vi "Scheduler.vi"(1 "RampRates":T1(array[cluster]), 3 "Room Temperature":dbl, 4 "CentigradeToFahrenheit":bool, 5 "error in (no error)":errorcluster, 6 "Action":dbl, 7 "Process_REF":string, 8 "State":dbl, 9 "Machine Settings":T2, 11 "Read File":string) -> (10 "Initialized":bool, 12 "Is Valid Schedule":bool, 13 "Waveform":waveform(dbl), 14 "Path Out":path, 15 "Setpoint Profile":cluster{"Time (s)":dbl, "setpoint (C)":dbl}[](array[cluster]), 17 "Sampling Rates":dbl[](array[numeric]), 18 "New RampRates":T1(array[cluster]), 19 "error out":errorcluster)   [LabVIEW 2018]
panel:
  out "Waveform Graph":waveform(dbl)(graph)
  in  "stop":bool
  in  "Path In":path
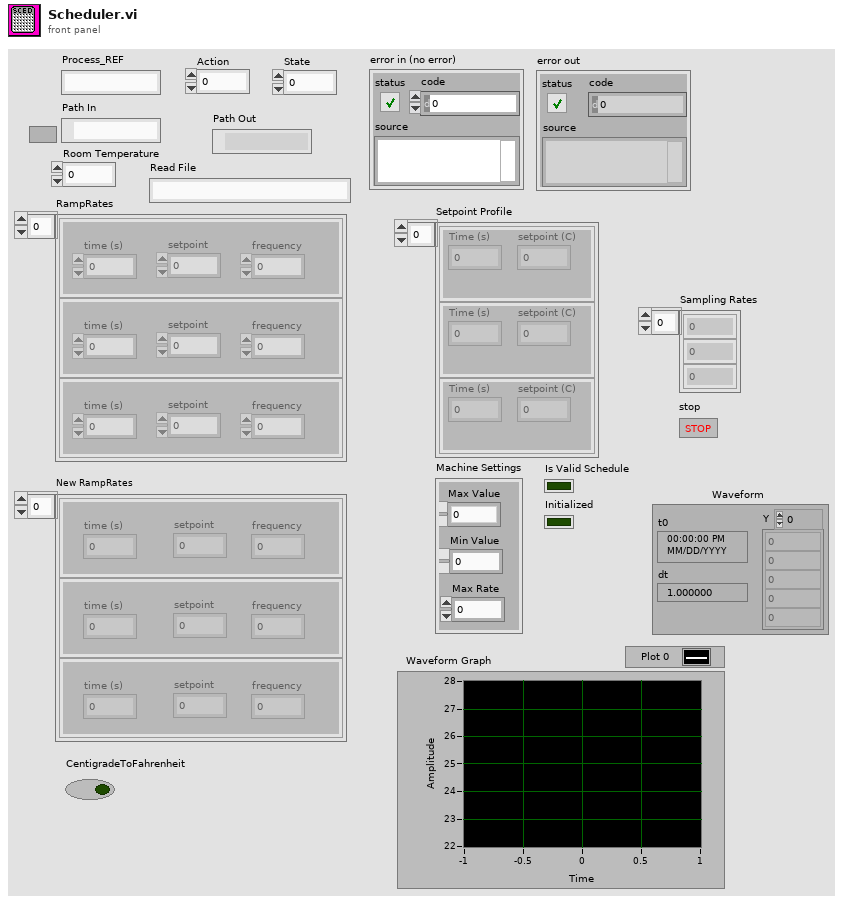
[diagram p1: front panel]
types:
  T1 = cluster{"time (s)":dbl, "setpoint ":dbl, "frequency":dbl}[]
  T2 = cluster{"Max Value":dbl, "Min Value":dbl, "Max Rate":dbl}
  T3 = cluster{"Duration (min)":dbl, "Rate (C/min) ":dbl, "Frequency (1/min)":dbl}[]
  T4 = cluster{"Duration (m)":dbl, "Rate (C/min)":dbl}[]
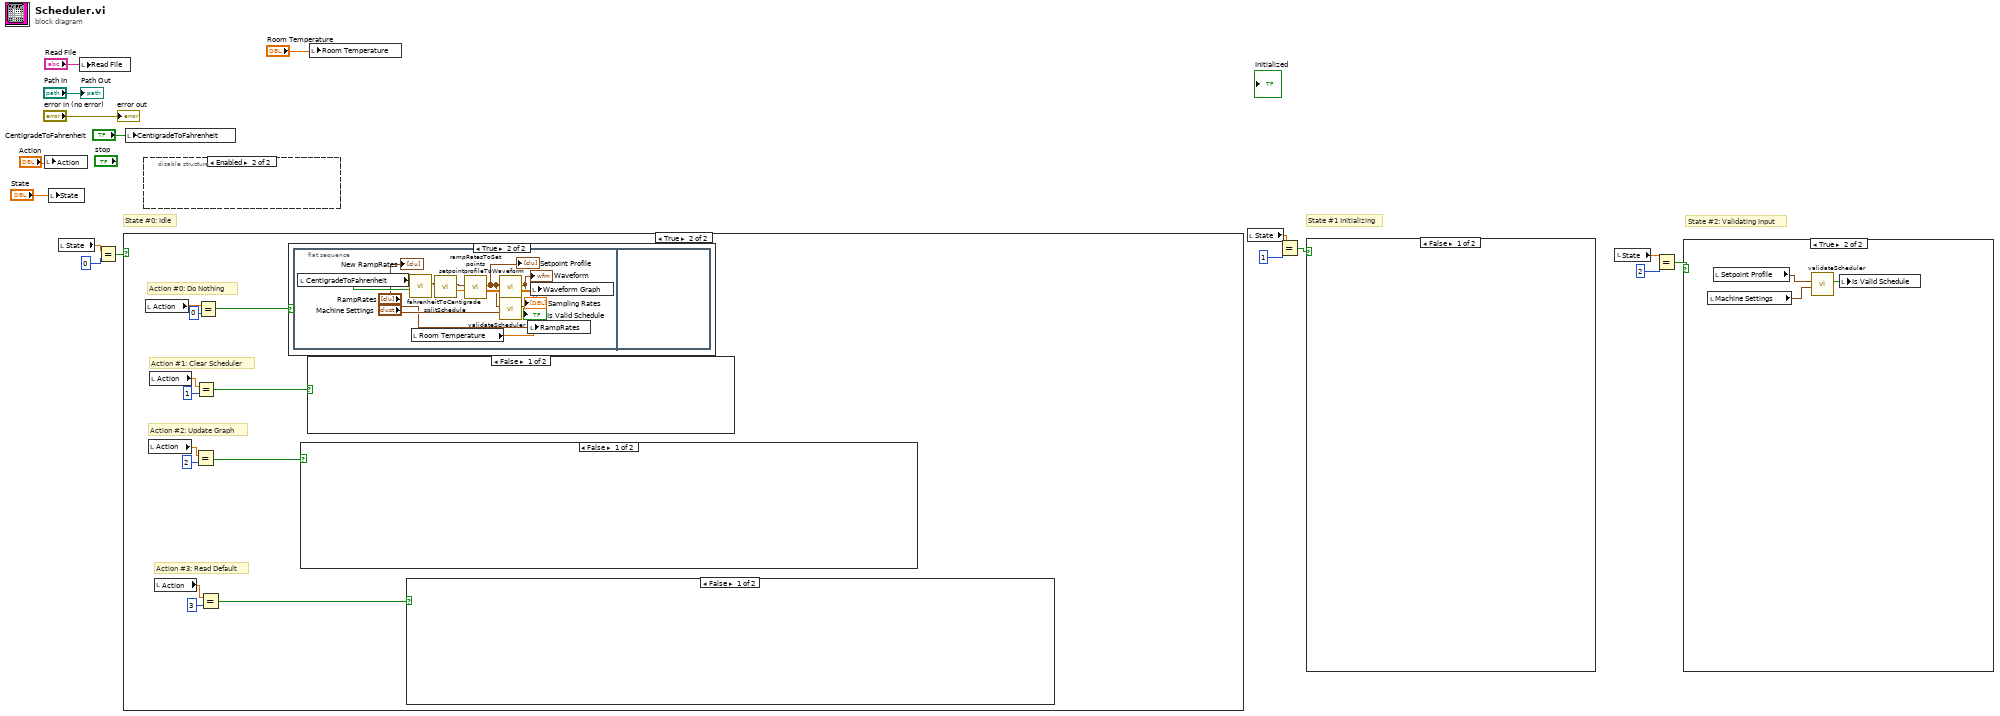
[diagram p0: block diagram]
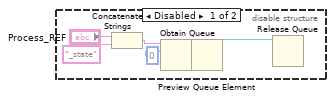
[diagram p2: hidden frame]
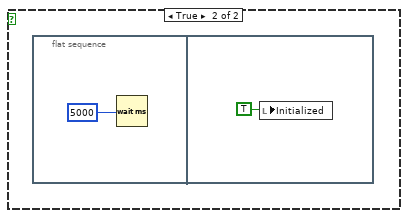
[diagram p4: hidden frame]
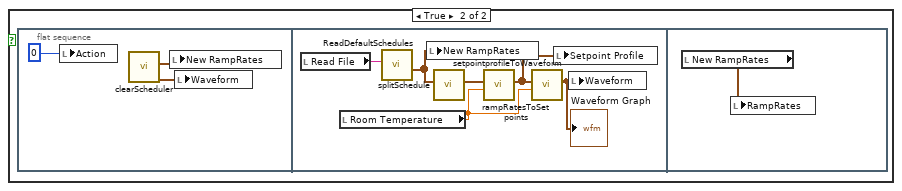
[diagram p7: hidden frame]
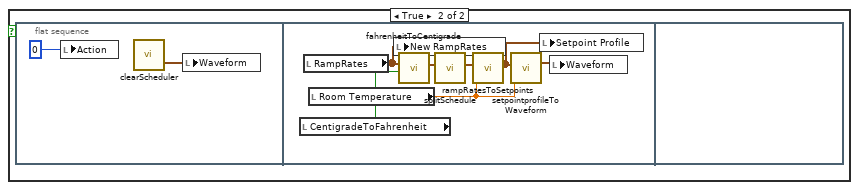
[diagram p8: hidden frame]
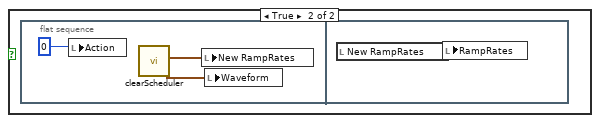
[diagram p9: hidden frame]
diagram:
  # "State #2: Validating Input"
  # "State #1 Initializing"
  # "State #0: Idle"
  n1 = local write "Action"("Action") -> ()
  n2 = local write "State"("State") -> ()
  n3 = local read "State"() -> (w11:dbl)
  n4 = local write "Read File"("Read File") -> ()
  n5 = Equal?(x=w11, y=0) -> (x = y?=w9:bool)
  n6 = case shown="True" w9 {
    frame False {
    }
    frame True {
      # "Action #0: Do Nothing"
      # "Action #3: Read Default"
      # "Action #2: Update Graph"
      # "Action #1: Clear Scheduler"
      n7 = local read "Action"() -> (w18:dbl)
      n8 = local read "Action"() -> (w24:dbl)
      n9 = local read "Action"() -> (w27:dbl)
      n10 = local read "Action"() -> (w21:dbl)
      n11 = Equal?(x=w24, y=2) -> (x = y?=w23:bool)
      n12 = Equal?(x=w27, y=1) -> (x = y?=w26:bool)
      n13 = Equal?(x=w18, y=0) -> (x = y?=w17:bool)
      n14 = Equal?(x=w21, y=3) -> (x = y?=w20:bool)
      n15 = case shown="True" w17 {
        frame False {
        }
        frame True {
          n16 = flat-sequence {
            frame #0 {
              n17 = local read "CentigradeToFahrenheit"() -> (w32:bool)
              n18 = call "fahrenheitToCentigrade.vi"("Convert?"=w32, "Schedule Before"="RampRates") -> ("Schedule After"=w33:T3)  [unwired: 9 in]
              n19 = local read "Room Temperature"() -> (w38:dbl)
              n20 = call "splitSchedule.vi"("Schedule"=w33) -> ("Sampling Rates"=→"Sampling Rates":dbl[], "Ramp Rates"=w36:T4)  [unwired: 9 in]
              n21 = call "rampRatesToSetpoints.vi"("Room Temperature"=w38, "Ramp Rates"=w36) -> ("Setpoint Profile"=w29:cluster{"Time (s)":dbl, "Setpoint (C)":dbl}[])  [unwired: 9 in]
              "Setpoint Profile" <- w29
              n22 = call "setpointprofileToWaveform.vi"("Room Temp Offset"=w38, "setpoint profile"=w29) -> ("Waveform"=w30:waveform(dbl))  [unwired: 9 in]
              "Waveform" <- w30
              n23 = call "validateScheduler.vi"("Constraints"="Machine Settings", "Schedule"=w29) -> ("Valid Input"=→"Is Valid Schedule":bool)  [unwired: 8 in, 1 out]
              n24 = local write "RampRates"("RampRates") -> ()
              n25 = local write "Waveform Graph"(w30) -> ()
              "New RampRates" <- "RampRates"
            }
            frame #1 {
            }
          }
        }
      }
      n26 = case shown="False" w23 {
        frame False {
        }
        frame True {
          n27 = flat-sequence {
            frame #0 {
              n28 = local write "Action"(0) -> ()
              n29 = call "clearScheduler.vi"() -> ("Empty Waveform"=w49:waveform(dbl))  [unwired: 8 in, 2 out]
              n30 = local write "Waveform"(w49) -> ()
            }
            frame #1 {
              n31 = local read "CentigradeToFahrenheit"() -> (w51:bool)
              n32 = local read "RampRates"() -> (w53:T1)
              n33 = local read "Room Temperature"() -> (w54:dbl)
              n34 = local write "New RampRates"(w53) -> ()
              n35 = call "fahrenheitToCentigrade.vi"("Convert?"=w51, "Schedule Before"=w53) -> ("Schedule After"=w57:T3)  [unwired: 9 in]
              n36 = call "splitSchedule.vi"("Schedule"=w57) -> ("Ramp Rates"=w55:T4)  [unwired: 9 in, 1 out]
              n37 = call "rampRatesToSetpoints.vi"("Room Temperature"=w54, "Ramp Rates"=w55) -> ("Setpoint Profile"=w52:cluster{"Time (s)":dbl, "Setpoint (C)":dbl}[])  [unwired: 9 in]
              n38 = call "setpointprofileToWaveform.vi"("Room Temp Offset"=w54, "setpoint profile"=w52) -> ("Waveform"=w56:waveform(dbl))  [unwired: 9 in]
              n39 = local write "Setpoint Profile"(w52) -> ()
              n40 = local write "Waveform"(w56) -> ()
            }
            frame #2 {
            }
          }
        }
      }
      n41 = case shown="False" w26 {
        frame False {
        }
        frame True {
          n42 = flat-sequence {
            frame #0 {
              n43 = local write "Action"(0) -> ()
              n44 = call "clearScheduler.vi"() -> ("Empty Waveform"=w58:waveform(dbl), "Empty Scheduler"=w59:T1)  [unwired: 8 in, 1 out]
              n45 = local write "New RampRates"(w59) -> ()
              n46 = local write "Waveform"(w58) -> ()
            }
            frame #1 {
              n47 = local read "New RampRates"() -> (w61:T1)
              n48 = local write "RampRates"(w61) -> ()
            }
          }
        }
      }
      n49 = case shown="False" w20 {
        frame False {
        }
        frame True {
          n50 = flat-sequence {
            frame #0 {
              n51 = local write "Action"(0) -> ()
              n52 = call "clearScheduler.vi"() -> ("Empty Waveform"=w39:waveform(dbl), "Empty Scheduler"=w40:T1)  [unwired: 8 in, 1 out]
              n53 = local write "New RampRates"(w40) -> ()
              n54 = local write "Waveform"(w39) -> ()
            }
            frame #1 {
              n55 = local read "Read File"() -> (w47:string)
              n56 = local read "Room Temperature"() -> (w43:dbl)
              n57 = call "ReadDefaultSchedules.vi"("File Name"=w47) -> ("Scheduler"=w46:T1)  [unwired: 8 in, 2 out]
              n58 = local write "New RampRates"(w46) -> ()
              n59 = call "splitSchedule.vi"("Schedule"=w46) -> ("Ramp Rates"=w44:T4)  [unwired: 9 in, 1 out]
              n60 = call "rampRatesToSetpoints.vi"("Room Temperature"=w43, "Ramp Rates"=w44) -> ("Setpoint Profile"=w42:cluster{"Time (s)":dbl, "Setpoint (C)":dbl}[])  [unwired: 9 in]
              n61 = call "setpointprofileToWaveform.vi"("Room Temp Offset"=w43, "setpoint profile"=w42) -> ("Waveform"=w45:waveform(dbl))  [unwired: 9 in]
              "Waveform Graph" <- w45
              n62 = local write "Setpoint Profile"(w42) -> ()
              n63 = local write "Waveform"(w45) -> ()
            }
            frame #2 {
              n64 = local read "New RampRates"() -> (w48:T1)
              n65 = local write "RampRates"(w48) -> ()
            }
          }
        }
      }
    }
  }
  n66 = local write "CentigradeToFahrenheit"("CentigradeToFahrenheit") -> ()
  n67 = disable-structure shown="Enabled" {
    frame Disabled {
      n68 = Concatenate Strings("Process_REF", "_state") -> (w64:string)
      n69 = Obtain Queue(name (unnamed)=w64, element data type=0) -> (queue out=w67:refnum<queue>)  [unwired: 3 in, 2 out]
      n70 = Preview Queue Element(queue=w67) -> (queue out=w62:refnum<queue>)  [unwired: 2 in, 3 out]
      n71 = Release Queue(queue=w62) -> ()  [unwired: 2 in, 3 out]
    }
    frame Enabled {
    }
  }
  n72 = local write "Room Temperature"("Room Temperature") -> ()
  n73 = local read "State"() -> (w7:dbl)
  n74 = Equal?(x=w7, y=1) -> (x = y?=w6:bool)
  n75 = case shown="False" w6 {
    frame False {
    }
    frame True {
      n76 = flat-sequence {
        frame #0 {
          n77 = Wait (ms)(milliseconds to wait=5000) -> ()  [unwired: 1 out]
        }
        frame #1 {
          n78 = local write "Initialized"(TRUE) -> ()
        }
      }
    }
  }
  n79 = local read "State"() -> (w3:dbl)
  n80 = Equal?(x=w3, y=2) -> (x = y?=w4:bool)
  n81 = case shown="True" w4 {
    frame False {
    }
    frame True {
      n82 = local read "Machine Settings"() -> (w72:T2)
      n83 = local read "Setpoint Profile"() -> (w70:cluster{"Time (s)":dbl, "setpoint (C)":dbl}[])
      n84 = call "validateScheduler.vi"("Constraints"=w72, "Schedule"=w70) -> ("Valid Input"=w71:bool)  [unwired: 8 in, 1 out]
      n85 = local write "Is Valid Schedule"(w71) -> ()
    }
  }
  "error out" <- "error in (no error)"
  "Path Out" <- "Path In"
